vi "Example CaseStructure 4.vi"(8 "Error In":errorcluster) -> (0 "Error Out":errorcluster, 1 "signal out":waveform(dbl), 3 "appended array":waveform(dbl)[](array[waveform]))   [LabVIEW 2014]
uses:
  <vilib>/measure/NI_MABase.lvlib
panel:
  out "signal out 4":waveform(dbl)
  out "signal out 3":waveform(dbl)
  out "signal out 2":waveform(dbl)
  out "String":string
  in  "case string":string
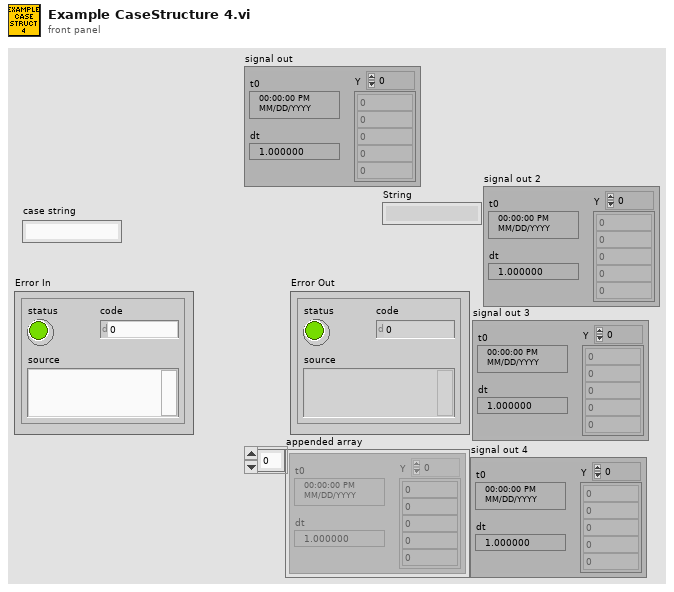
[diagram p1: front panel]
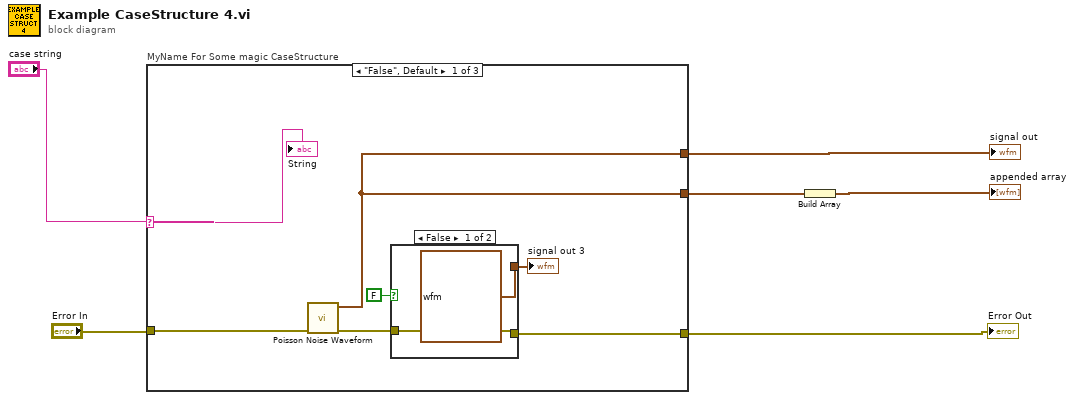
[diagram p0: block diagram]
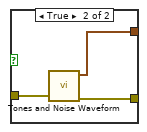
[diagram p2: hidden frame]
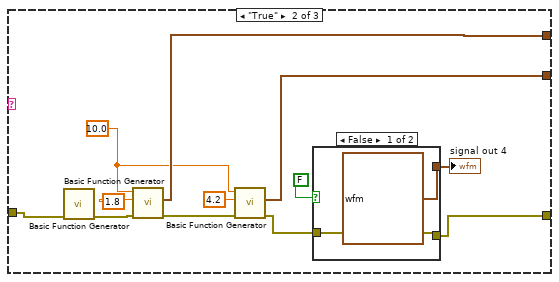
[diagram p3: hidden frame]
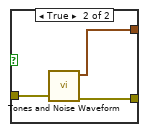
[diagram p4: hidden frame]
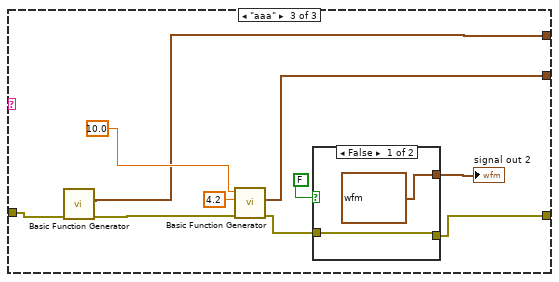
[diagram p5: hidden frame]
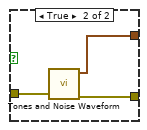
[diagram p6: hidden frame]
diagram:
  n1 = case "MyName For Some magic CaseStructure" shown="\"False\", Default" "case string" {
    selector: "case string" -> [w11 _ _]
    tunnel: "Error In" -> [w13 w21 w39]
    tunnel: [w9 w23 w40] -> w2
    tunnel: [w12 w28 w37] -> w5
    tunnel: [w12 w27 w44] -> w4
    frame "False", Default {
      n2 = call <vilib>:"Poisson Noise Waveform.vi"("error in (no error)"=w13) -> ("error out"=w10:errorcluster, "signal out"=w12:waveform(dbl))  [unwired: 9 in]
      n3 = case shown="False" FALSE {
        tunnel: w10 -> [w15 w18]
        tunnel: [w15 w17] -> w9
        tunnel: [waveform(dbl) {"t0"=timestamp(0 s since 1904-01-01), "dt"=1.0, "Y"=[]} ("signal out") w16] -> w7
        frame False {
        }
        frame True {
          n4 = call <vilib>:"Tones and Noise Waveform.vi"("error in (no error)"=w18) -> ("error out"=w17:errorcluster, "signal out"=w16:waveform(dbl))  [unwired: 9 in]
        }
      }
      "signal out 3" <- w7
      "String" <- w11
    }
    frame "True" {
      w26 = 10.0 ("frequency")
      n5 = call <vilib>:"Basic Function Generator.vi"("error in (no error)"=w21) -> ("error out"=w20:errorcluster)  [unwired: 8 in, 2 out]
      n6 = call <vilib>:"Basic Function Generator.vi"("error in (no error)"=w20, "amplitude"=1.8, "frequency"=w26) -> ("error out"=w30:errorcluster, "signal out"=w28:waveform(dbl))  [unwired: 6 in, 1 out]
      n7 = call <vilib>:"Basic Function Generator.vi"("error in (no error)"=w30, "amplitude"=4.2, "frequency"=w26) -> ("error out"=w24:errorcluster, "signal out"=w27:waveform(dbl))  [unwired: 6 in, 1 out]
      n8 = case shown="False" FALSE {
        tunnel: w24 -> [w32 w35]
        tunnel: [w32 w34] -> w23
        tunnel: [waveform(dbl) {"t0"=timestamp(0 s since 1904-01-01), "dt"=1.0, "Y"=[]} ("signal out") w33] -> w19
        frame False {
        }
        frame True {
          n9 = call <vilib>:"Tones and Noise Waveform.vi"("error in (no error)"=w35) -> ("error out"=w34:errorcluster, "signal out"=w33:waveform(dbl))  [unwired: 9 in]
        }
      }
      "signal out 4" <- w19
    }
    frame "aaa" {
      n10 = call <vilib>:"Basic Function Generator.vi"("error in (no error)"=w39) -> ("error out"=w38:errorcluster, "signal out"=w37:waveform(dbl))  [unwired: 8 in, 1 out]
      n11 = call <vilib>:"Basic Function Generator.vi"("error in (no error)"=w38, "amplitude"=4.2, "frequency"=10.0) -> ("error out"=w41:errorcluster, "signal out"=w44:waveform(dbl))  [unwired: 6 in, 1 out]
      n12 = case shown="False" FALSE {
        tunnel: w41 -> [w47 w50]
        tunnel: [w47 w49] -> w40
        tunnel: [waveform(dbl) {"t0"=timestamp(0 s since 1904-01-01), "dt"=1.0, "Y"=[]} ("signal out") w48] -> w36
        frame False {
        }
        frame True {
          n13 = call <vilib>:"Tones and Noise Waveform.vi"("error in (no error)"=w50) -> ("error out"=w49:errorcluster, "signal out"=w48:waveform(dbl))  [unwired: 9 in]
        }
      }
      "signal out 2" <- w36
    }
  }
  "Error Out" <- w2
  "signal out" <- w5
  n14 = Build Array(w4) -> (→"appended array":waveform(dbl)[])
